vi "Result_Test.vi"(8 "error in (no error)":errorcluster caption="entrée d'erreur (pas d'erreur)", 11 "Flash_Jlink en entrée":refnum<class "RSSI_Enocean.lvclass">) -> (0 "error out":errorcluster caption="sortie d'erreur", 3 "Flash_Jlink en sortie":refnum<class "RSSI_Enocean.lvclass">)   [LabVIEW 2020, in "Library Test.lvlib" / "RSSI_Enocean.lvclass"]
uses:
  RSSI_Enocean.lvclass
  C:/Users/ngarcin/OneDrive - Altyor/Standard TB/Suite TB45/Class/Test/Test (Default)/Test (Default).lvclass
  Commun VI/TypeDef/Variable Printable.ctl
  Test_Without_Instr/Test_Without_Inst.lvclass
  Commun VI/Library Commun.lvlib
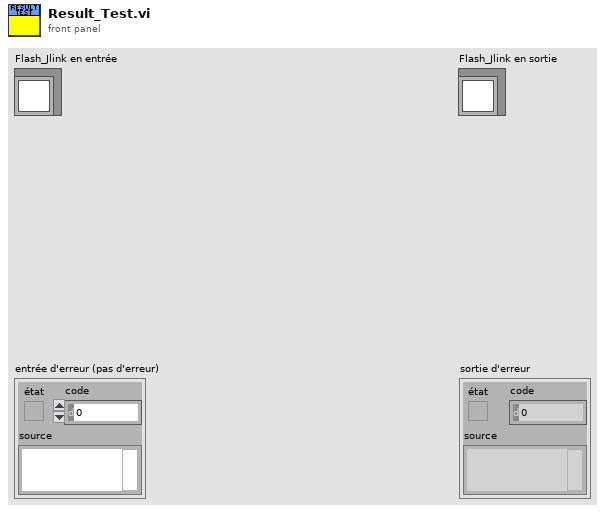
[diagram p1: front panel]
types:
  T1 = enum16{"Get Variable", "Get All Variables", "Set Variable", "Delete Variable", "Delete All Variable"}
  T2 = typedef "Variable Printable.ctl" = string
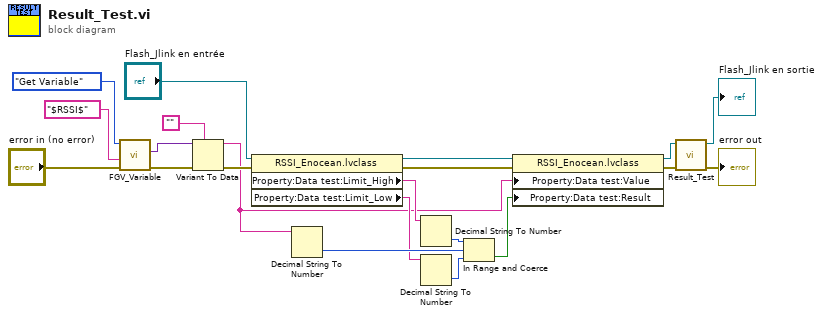
[diagram p0: block diagram]
diagram:
  n1 = call "FGV_Variable.vi"("error in (no error)"="error in (no error)", "Variable"=T2 "$RSSI$", "Function"=T1."Get Variable") -> ("error out"=w14:errorcluster, "Data Out"=w13:variant)  [unwired: 6 in, 1 out]
  n2 = Variant To Data(error in=w14, type="", Variant=w13) -> (data=w1:string, error out=w11:errorcluster)
  n3 = property class="RSSI_Enocean.lvclass"(reference="Flash_Jlink en entrée", error in=w11) -> (reference out=w8:refnum<class "RSSI_Enocean.lvclass">, error out=w10:errorcluster, "Property:Data test:Limit_High"=w4:string, "Property:Data test:Limit_Low"=w3:string)
  n4 = Decimal String To Number(string=w1) -> (number=w6:i32)  [unwired: 2 in, 1 out]
  n5 = Decimal String To Number(string=w4) -> (number=w7:i32)  [unwired: 2 in, 1 out]
  n6 = Decimal String To Number(string=w3) -> (number=w5:i32)  [unwired: 2 in, 1 out]
  n7 = In Range and Coerce(upper limit=w7, x=w6, lower limit=w5) -> (In Range?=w2:bool)  [unwired: 1 out]
  n8 = property class="RSSI_Enocean.lvclass"(reference=w8, error in=w10, "Property:Data test:Value"=w1, "Property:Data test:Result"=w2) -> (reference out=w18:refnum<class "RSSI_Enocean.lvclass">, error out=w19:errorcluster)
  n9 = call-parent "Result_Test.vi"("error in (no error)"=w19, "Test_Without_Inst en entrée"=w18) -> ("error out"=→"error out":errorcluster, "Test_Without_Inst en sortie"=→"Flash_Jlink en sortie":refnum<class "RSSI_Enocean.lvclass">)  [unwired: 8 in]
